vi "GetQueueName.vi"(11 "QueueIn":refnum<queue>) -> (3 "String":string)   [LabVIEW 2021, in "YActor.lvclass"]
uses:
  YActor.lvclass
  CmdCtrl.ctl
  AsyncErrorHandling.ctl
  CallMode.ctl
  YActor.lvclass/YActor.ctl
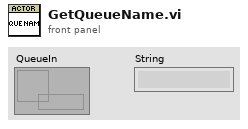
[diagram p1: front panel]
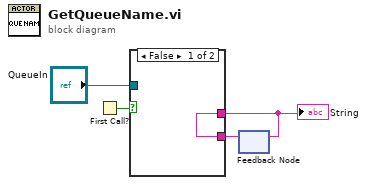
[diagram p0: block diagram]
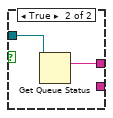
[diagram p2: hidden frame]
diagram:
  n1 = First Call?() -> (First Call?: T/F=w3:bool)
  n2 = feedback #1() -> (w1:string)  [unwired: 1 in]
  n3 = case shown="False" w3 {
    tunnel: [w5 w7] -> w2
    tunnel: "QueueIn" -> [_ w6]
    tunnel: w1 -> [w5 _]
    frame False {
    }
    frame True {
      n4 = Get Queue Status(queue=w6) -> (queue name=w7:string)  [unwired: 2 in, 7 out]
    }
  }
  "String" <- w2
  n5 = feedback-in #1(w2) -> ()
